vi "Set Voltage.vi"(8 "error in":errorcluster, 10 "Voltage":dbl) -> (0 "error out":errorcluster)   [LabVIEW 2021, in "PS.lvlib"]
doc: "_____\nCreated using DQMH Event Scripter 6.0.0.122."
uses:
  PS.lvlib
  Set Voltage Argument--cluster.ctl
  <vilib>/DQMH Consortium/Lumos API/Libraries/SDV API/SDV API.lvlib
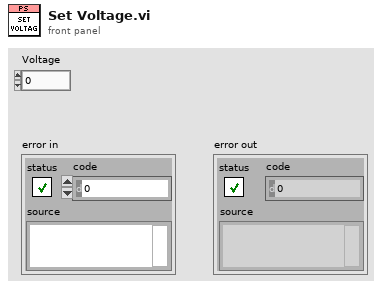
[diagram p1: front panel]
types:
  T1 = typedef "PS.lvlib/Set Voltage Argument--cluster.ctl" = cluster{"Voltage":dbl}
  T2 = typedef "PS.lvlib/Request Events--cluster.ctl" = cluster{"Stop Module":refnum<user-event>, "Show Panel":refnum<user-event>, "Hide Panel":refnum<user-event>, "Get Module Execution Status":refnum<user-event>, "Show Diagram":refnum<user-event>, "Set Power Supply":refnum<user-event>, "Set Voltage":refnum<user-event>, "Set Current":refnum<user-event>, "Set Output":refnum<user-event>, "Open":refnum<user-event>, "Close":refnum<user-event>, "Get PS Data":refnum<user-event>, "Load in SubPane":refnum<user-event>, "UnLoad SubPane":refnum<user-event>}
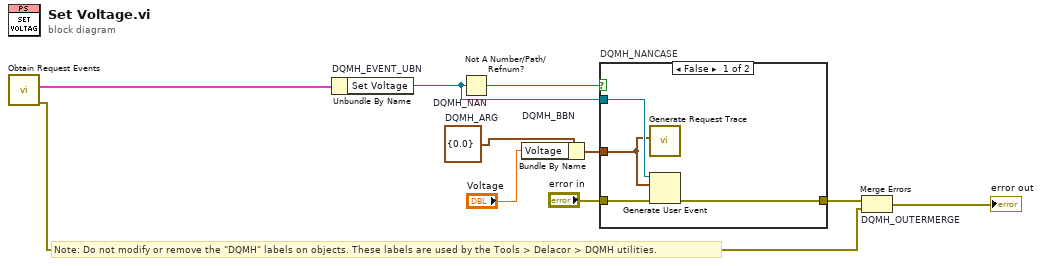
[diagram p0: block diagram]
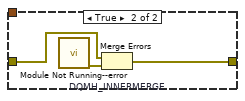
[diagram p2: hidden frame]
diagram:
  w4 = T1 {"Voltage"=0.0}  # DQMH_ARG
  # "Note: Do not modify or remove the \"DQMH\" labels on objects. These labels are used by the Tools > Delacor > DQMH utilities."
  n1 = call "Obtain Request Events.vi"() -> ("error out"=w2:errorcluster, "PS Request Events"=w1:T2)  [unwired: 10 in]
  n2 = Unbundle By Name "DQMH_EVENT_UBN"(w1) -> ("Set Voltage"=w6:refnum<user-event>)
  n3 = Not A Number/Path/Refnum? "DQMH_NAN"(number/path/refnum=w6) -> (NaN/Path/Refnum?=w7:bool)
  n4 = Bundle By Name "DQMH_BBN"(cluster=w4, "Voltage"="Voltage") -> (w8:T1)
  n5 = case "DQMH_NANCASE" shown="False" w7 {
    tunnel: "error in" -> [w14 w17]
    tunnel: [w13 w16] -> w5
    tunnel: w6 -> [w12 _]
    tunnel: w8 -> [w11 _]
    frame False {
      n6 = call <vilib>:"Generate Request Trace.vi"("Payload"=w11) -> ()  [unwired: 10 in, 1 out]
      n7 = Generate User Event(user event=w12, event data cluster=w11, error in=w14) -> (error out=w13:errorcluster)  [unwired: 1 in, 1 out]
    }
    frame True {
      n8 = call "Module Not Running--error.vi"() -> ("error out"=w15:errorcluster)  [unwired: 11 in]
      n9 = Merge Errors "DQMH_INNERMERGE"(w17, w15) -> (w16:errorcluster)
    }
  }
  n10 = Merge Errors "DQMH_OUTERMERGE"(w5, w2) -> (→"error out":errorcluster)
